vi "Agitator Loop.vi"(8 "error in (no error)":errorcluster) -> (0 "error out":errorcluster)   [LabVIEW 2021]
uses:
  Global Variables/RT GV.vi
panel:
  in  "Stop":bool
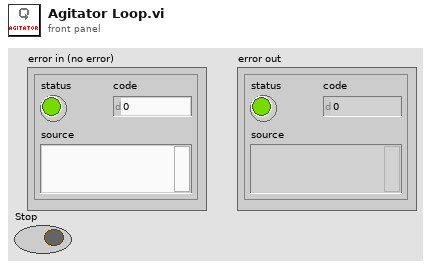
[diagram p1: front panel]
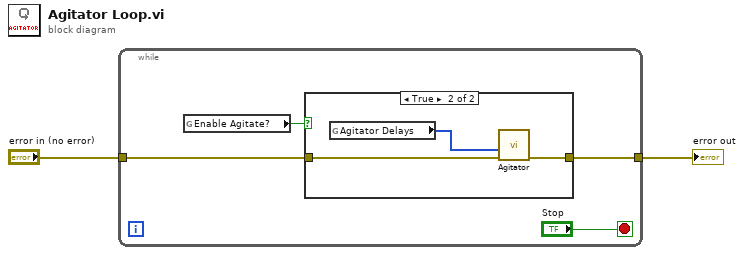
[diagram p0: block diagram]
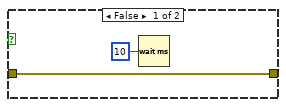
[diagram p2: hidden frame]
diagram:
  n1 = while {
    tunnel: "error in (no error)" -> [w6]
    tunnel: [w4] -> w1
    stop <- "Stop" stop-if-true
    n2 = global read "RT GV.vi" "Enable Agitate?"() -> (w5:bool)
    n3 = case shown="True" w5 {
      tunnel: w6 -> [w8 w11]
      tunnel: [w8 w10] -> w4
      frame False {
        n4 = Wait (ms)(milliseconds to wait=u32 10) -> ()  [unwired: 1 out]
      }
      frame True {
        n5 = global read "RT GV.vi" "Agitator Delays"() -> (w9:u32[])
        n6 = call "Agitator.vi"("error in (no error)"=w11, "Agitator Delays"=w9) -> ("error out"=w10:errorcluster)  [unwired: 8 in, 1 out]
      }
    }
  }
  "error out" <- w1
